vi "App - analyze RUS V6.vi"() -> ()   [LabVIEW 2018] (continued)
"file format"=enum."binary", "power(V)"=2.1, "Magn Field(T) "=0.0}, {"temperature"=20.054, "temperature str"="20.05400", "file path"=path "D:/Data/Ultrasound/LSCO/LSCO22__130814c/5_Cooling_2nd_try/September_2014/091714/20.05400K_500_2500_2.10000V_0.00000T_Sep17-2014__19-47-23_001_091714.bin", "last mod"=timestamp(3493842443 s since 1904-01-01), "file name str"="D:\\Data\\Ultrasound\\LSCO\\LSCO22__130814c\\5_Cooling_2nd_try\\September_2014\\091714\\20.05400K_500_2500_2.10000V_0.00000T_Sep17-2014__19-47-23_001_091714.bin", "mod time(min)"=58230707.38333333, "file format"=enum."binary", "power(V)"=2.1, "Magn Field(T) "=0.0}, {"temperature"=19.964, "temperature str"="19.96400", "file path"=path "D:/Data/Ultrasound/LSCO/LSCO22__130814c/5_Cooling_2nd_try/September_2014/091714/19.96400K_500_2500_2.10000V_0.00000T_Sep17-2014__19-48-42_001_091714.bin", "last mod"=timestamp(3493842522 s since 1904-01-01), "file name str"="D:\\Data\\Ultrasound\\LSCO\\LSCO22__130814c\\5_Cooling_2nd_try\\September_2014\\091714\\19.96400K_500_2500_2.10000V_0.00000T_Sep17-2014__19-48-42_001_091714.bin", "mod time(min)"=58230708.7, "file format"=enum."binary", "power(V)"=2.1, "Magn Field(T) "=0.0}, {"temperature"=19.857, "temperature str"="19.85700", "file path"=path "D:/Data/Ultrasound/LSCO/LSCO22__130814c/5_Cooling_2nd_try/September_2014/091714/19.85700K_500_2500_2.10000V_0.00000T_Sep17-2014__19-50-02_001_091714.bin", "last mod"=timestamp(3493842602 s since 1904-01-01), "file name str"="D:\\Data\\Ultrasound\\LSCO\\LSCO22__130814c\\5_Cooling_2nd_try\\September_2014\\091714\\19.85700K_500_2500_2.10000V_0.00000T_Sep17-2014__19-50-02_001_091714.bin", "mod time(min)"=58230710.03333333, "file format"=enum."binary", "power(V)"=2.1, "Magn Field(T) "=0.0}, {"temperature"=19.754, "temperature str"="19.75400", "file path"=path "D:/Data/Ultrasound/LSCO/LSCO22__130814c/5_Cooling_2nd_try/September_2014/091714/19.75400K_500_2500_2.10000V_0.00000T_Sep17-2014__19-51-21_001_091714.bin", "last mod"=timestamp(3493842681 s since 1904-01-01), "file name str"="D:\\Data\\Ultrasound\\LSCO\\LSCO22__130814c\\5_Cooling_2nd_try\\September_2014\\091714\\19.75400K_500_2500_2.10000V_0.00000T_Sep17-2014__19-51-21_001_091714.bin", "mod time(min)"=58230711.35, "file format"=enum."binary", "power(V)"=2.1, "Magn Field(T) "=0.0}, {"temperature"=19.658, "temperature str"="19.65800", "file path"=path "D:/Data/Ultrasound/LSCO/LSCO22__130814c/5_Cooling_2nd_try/September_2014/091714/19.65800K_500_2500_2.10000V_0.00000T_Sep17-2014__19-52-41_001_091714.bin", "last mod"=timestamp(3493842761 s since 1904-01-01), "file name str"="D:\\Data\\Ultrasound\\LSCO\\LSCO22__130814c\\5_Cooling_2nd_try\\September_2014\\091714\\19.65800K_500_2500_2.10000V_0.00000T_Sep17-2014__19-52-41_001_091714.bin", "mod time(min)"=58230712.68333333, "file format"=enum."binary", "power(V)"=2.1, "Magn Field(T) "=0.0}, {"temperature"=19.556, "temperature str"="19.55600", "file path"=path "D:/Data/Ultrasound/LSCO/LSCO22__130814c/5_Cooling_2nd_try/September_2014/091714/19.55600K_500_2500_2.10000V_0.00000T_Sep17-2014__19-54-00_001_091714.bin", "last mod"=timestamp(3493842840 s since 1904-01-01), "file name str"="D:\\Data\\Ultrasound\\LSCO\\LSCO22__130814c\\5_Cooling_2nd_try\\September_2014\\091714\\19.55600K_500_2500_2.10000V_0.00000T_Sep17-2014__19-54-00_001_091714.bin", "mod time(min)"=58230714.0, "file format"=enum."binary", "power(V)"=2.1, "Magn Field(T) "=0.0}, {"temperature"=19.452, "temperature str"="19.45200", "file path"=path "D:/Data/Ultrasound/LSCO/LSCO22__130814c/5_Cooling_2nd_try/September_2014/091714/19.45200K_500_2500_2.10000V_0.00000T_Sep17-2014__19-55-19_001_091714.bin", "last mod"=timestamp(3493842919 s since 1904-01-01), "file name str"="D:\\Data\\Ultrasound\\LSCO\\LSCO22__130814c\\5_Cooling_2nd_try\\September_2014\\091714\\19.45200K_500_2500_2.10000V_0.00000T_Sep17-2014__19-55-19_001_091714.bin", "mod time(min)"=58230715.31666667, "file format"=enum."binary", "power(V)"=2.1, "Magn Field(T) "=0.0}, {"temperature"=19.356, "temperature str"="19.35600", "file path"=path "D:/Data/Ultrasound/LSCO/LSCO22__130814c/5_Cooling_2nd_try/September_2014/091714/19.35600K_500_2500_2.10000V_0.00000T_Sep17-2014__19-56-39_001_091714.bin", "last mod"=timestamp(3493842999 s since 1904-01-01), "file name str"="D:\\Data\\Ultrasound\\LSCO\\LSCO22__130814c\\5_Cooling_2nd_try\\September_2014\\091714\\19.35600K_500_2500_2.10000V_0.00000T_Sep17-2014__19-56-39_001_091714.bin", "mod time(min)"=58230716.65, "file format"=enum."binary", "power(V)"=2.1, "Magn Field(T) "=0.0}, {"temperature"=19.258, "temperature str"="19.25800", "file path"=path "D:/Data/Ultrasound/LSCO/LSCO22__130814c/5_Cooling_2nd_try/September_2014/091714/19.25800K_500_2500_2.10000V_0.00000T_Sep17-2014__19-57-58_001_091714.bin", "last mod"=timestamp(3493843078 s since 1904-01-01), "file name str"="D:\\Data\\Ultrasound\\LSCO\\LSCO22__130814c\\5_Cooling_2nd_try\\September_2014\\091714\\19.25800K_500_2500_2.10000V_0.00000T_Sep17-2014__19-57-58_001_091714.bin", "mod time(min)"=58230717.96666667, "file format"=enum."binary", "power(V)"=2.1, "Magn Field(T) "=0.0}, {"temperature"=19.154, "temperature str"="19.15400", "file path"=path "D:/Data/Ultrasound/LSCO/LSCO22__130814c/5_Cooling_2nd_try/September_2014/091714/19.15400K_500_2500_2.10000V_0.00000T_Sep17-2014__19-59-17_001_091714.bin", "last mod"=timestamp(3493843157 s since 1904-01-01), "file name str"="D:\\Data\\Ultrasound\\LSCO\\LSCO22__130814c\\5_Cooling_2nd_try\\September_2014\\091714\\19.15400K_500_2500_2.10000V_0.00000T_Sep17-2014__19-59-17_001_091714.bin", "mod time(min)"=58230719.28333333, "file format"=enum."binary", "power(V)"=2.1, "Magn Field(T) "=0.0}, {"temperature"=19.054, "temperature str"="19.05400", "file path"=path "D:/Data/Ultrasound/LSCO/LSCO22__130814c/5_Cooling_2nd_try/September_2014/091714/19.05400K_500_2500_2.10000V_0.00000T_Sep17-2014__20-00-37_001_091714.bin", "last mod"=timestamp(3493843237 s since 1904-01-01), "file name str"="D:\\Data\\Ultrasound\\LSCO\\LSCO22__130814c\\5_Cooling_2nd_try\\September_2014\\091714\\19.05400K_500_2500_2.10000V_0.00000T_Sep17-2014__20-00-37_001_091714.bin", "mod time(min)"=58230720.61666667, "file format"=enum."binary", "power(V)"=2.1, "Magn Field(T) "=0.0}, {"temperature"=18.951, "temperature str"="18.95100", "file path"=path "D:/Data/Ultrasound/LSCO/LSCO22__130814c/5_Cooling_2nd_try/September_2014/091714/18.95100K_500_2500_2.10000V_0.00000T_Sep17-2014__20-01-56_001_091714.bin", "last mod"=timestamp(3493843316 s since 1904-01-01), "file name str"="D:\\Data\\Ultrasound\\LSCO\\LSCO22__130814c\\5_Cooling_2nd_try\\September_2014\\091714\\18.95100K_500_2500_2.10000V_0.00000T_Sep17-2014__20-01-56_001_091714.bin", "mod time(min)"=58230721.93333333, "file format"=enum."binary", "power(V)"=2.1, "Magn Field(T) "=0.0}, {"temperature"=18.852, "temperature str"="18.85200", "file path"=path "D:/Data/Ultrasound/LSCO/LSCO22__130814c/5_Cooling_2nd_try/September_2014/091714/18.85200K_500_2500_2.10000V_0.00000T_Sep17-2014__20-03-16_001_091714.bin", "last mod"=timestamp(3493843396 s since 1904-01-01), "file name str"="D:\\Data\\Ultrasound\\LSCO\\LSCO22__130814c\\5_Cooling_2nd_try\\September_2014\\091714\\18.85200K_500_2500_2.10000V_0.00000T_Sep17-2014__20-03-16_001_091714.bin", "mod time(min)"=58230723.266666666, "file format"=enum."binary", "power(V)"=2.1, "Magn Field(T) "=0.0}, {"temperature"=18.757, "temperature str"="18.75700", "file path"=path "D:/Data/Ultrasound/LSCO/LSCO22__130814c/5_Cooling_2nd_try/September_2014/091714/18.75700K_500_2500_2.10000V_0.00000T_Sep17-2014__20-04-35_001_091714.bin", "last mod"=timestamp(3493843475 s since 1904-01-01), "file name str"="D:\\Data\\Ultrasound\\LSCO\\LSCO22__130814c\\5_Cooling_2nd_try\\September_2014\\091714\\18.75700K_500_2500_2.10000V_0.00000T_Sep17-2014__20-04-35_001_091714.bin", "mod time(min)"=58230724.583333336, "file format"=enum."binary", "power(V)"=2.1, "Magn Field(T) "=0.0}, {"temperature"=18.649, "temperature str"="18.64900", "file path"=path "D:/Data/Ultrasound/LSCO/LSCO22__130814c/5_Cooling_2nd_try/September_2014/091714/18.64900K_500_2500_2.10000V_0.00000T_Sep17-2014__20-05-54_001_091714.bin", "last mod"=timestamp(3493843554 s since 1904-01-01), "file name str"="D:\\Data\\Ultrasound\\LSCO\\LSCO22__130814c\\5_Cooling_2nd_try\\September_2014\\091714\\18.64900K_500_2500_2.10000V_0.00000T_Sep17-2014__20-05-54_001_091714.bin", "mod time(min)"=58230725.9, "file format"=enum."binary", "power(V)"=2.1, "Magn Field(T) "=0.0}, {"temperature"=18.548, "temperature str"="18.54800", "file path"=path "D:/Data/Ultrasound/LSCO/LSCO22__130814c/5_Cooling_2nd_try/September_2014/091714/18.54800K_500_2500_2.10000V_0.00000T_Sep17-2014__20-07-14_001_091714.bin", "last mod"=timestamp(3493843634 s since 1904-01-01), "file name str"="D:\\Data\\Ultrasound\\LSCO\\LSCO22__130814c\\5_Cooling_2nd_try\\September_2014\\091714\\18.54800K_500_2500_2.10000V_0.00000T_Sep17-2014__20-07-14_001_091714.bin", "mod time(min)"=58230727.233333334, "file format"=enum."binary", "power(V)"=2.1, "Magn Field(T) "=0.0}, {"temperature"=18.451, "temperature str"="18.45100", "file path"=path "D:/Data/Ultrasound/LSCO/LSCO22__130814c/5_Cooling_2nd_try/September_2014/091714/18.45100K_500_2500_2.10000V_0.00000T_Sep17-2014__20-08-33_001_091714.bin", "last mod"=timestamp(3493843713 s since 1904-01-01), "file name str"="D:\\Data\\Ultrasound\\LSCO\\LSCO22__130814c\\5_Cooling_2nd_try\\September_2014\\091714\\18.45100K_500_2500_2.10000V_0.00000T_Sep17-2014__20-08-33_001_091714.bin", "mod time(min)"=58230728.55, "file format"=enum."binary", "power(V)"=2.1, "Magn Field(T) "=0.0}, {"temperature"=18.346, "temperature str"="18.34600", "file path"=path "D:/Data/Ultrasound/LSCO/LSCO22__130814c/5_Cooling_2nd_try/September_2014/091714/18.34600K_500_2500_2.10000V_0.00000T_Sep17-2014__20-09-53_001_091714.bin", "last mod"=timestamp(3493843793 s since 1904-01-01), "file name str"="D:\\Data\\Ultrasound\\LSCO\\LSCO22__130814c\\5_Cooling_2nd_try\\September_2014\\091714\\18.34600K_500_2500_2.10000V_0.00000T_Sep17-2014__20-09-53_001_091714.bin", "mod time(min)"=58230729.88333333, "file format"=enum."binary", "power(V)"=2.1, "Magn Field(T) "=0.0}, {"temperature"=18.245, "temperature str"="18.24500", "file path"=path "D:/Data/Ultrasound/LSCO/LSCO22__130814c/5_Cooling_2nd_try/September_2014/091714/18.24500K_500_2500_2.10000V_0.00000T_Sep17-2014__20-11-12_001_091714.bin", "last mod"=timestamp(3493843872 s since 1904-01-01), "file name str"="D:\\Data\\Ultrasound\\LSCO\\LSCO22__130814c\\5_Cooling_2nd_try\\September_2014\\091714\\18.24500K_500_2500_2.10000V_0.00000T_Sep17-2014__20-11-12_001_091714.bin", "mod time(min)"=58230731.2, "file format"=enum."binary", "power(V)"=2.1, "Magn Field(T) "=0.0}, {"temperature"=18.147, "temperature str"="18.14700", "file path"=path "D:/Data/Ultrasound/LSCO/LSCO22__130814c/5_Cooling_2nd_try/September_2014/091714/18.14700K_500_2500_2.10000V_0.00000T_Sep17-2014__20-12-31_001_091714.bin", "last mod"=timestamp(3493843951 s since 1904-01-01), "file name str"="D:\\Data\\Ultrasound\\LSCO\\LSCO22__130814c\\5_Cooling_2nd_try\\September_2014\\091714\\18.14700K_500_2500_2.10000V_0.00000T_Sep17-2014__20-12-31_001_091714.bin", "mod time(min)"=58230732.516666666, "file format"=enum."binary", "power(V)"=2.1, "Magn Field(T) "=0.0}, {"temperature"=18.042, "temperature str"="18.04200", "file path"=path "D:/Data/Ultrasound/LSCO/LSCO22__130814c/5_Cooling_2nd_try/September_2014/091714/18.04200K_500_2500_2.10000V_0.00000T_Sep17-2014__20-13-51_001_091714.bin", "last mod"=timestamp(3493844031 s since 1904-01-01), "file name str"="D:\\Data\\Ultrasound\\LSCO\\LSCO22__130814c\\5_Cooling_2nd_try\\September_2014\\091714\\18.04200K_500_2500_2.10000V_0.00000T_Sep17-2014__20-13-51_001_091714.bin", "mod time(min)"=58230733.85, "file format"=enum."binary", "power(V)"=2.1, "Magn Field(T) "=0.0}, {"temperature"=17.951, "temperature str"="17.95100", "file path"=path "D:/Data/Ultrasound/LSCO/LSCO22__130814c/5_Cooling_2nd_try/September_2014/091714/17.95100K_500_2500_2.10000V_0.00000T_Sep17-2014__20-15-10_001_091714.bin", "last mod"=timestamp(3493844110 s since 1904-01-01), "file name str"="D:\\Data\\Ultrasound\\LSCO\\LSCO22__130814c\\5_Cooling_2nd_try\\September_2014\\091714\\17.95100K_500_2500_2.10000V_0.00000T_Sep17-2014__20-15-10_001_091714.bin", "mod time(min)"=58230735.166666664, "file format"=enum."binary", "power(V)"=2.1, "Magn Field(T) "=0.0}, {"temperature"=17.844, "temperature str"="17.84400", "file path"=path "D:/Data/Ultrasound/LSCO/LSCO22__130814c/5_Cooling_2nd_try/September_2014/091714/17.84400K_500_2500_2.10000V_0.00000T_Sep17-2014__20-16-29_001_091714.bin", "last mod"=timestamp(3493844189 s since 1904-01-01), "file name str"="D:\\Data\\Ultrasound\\LSCO\\LSCO22__130814c\\5_Cooling_2nd_try\\September_2014\\091714\\17.84400K_500_2500_2.10000V_0.00000T_Sep17-2014__20-16-29_001_091714.bin", "mod time(min)"=58230736.483333334, "file format"=enum."binary", "power(V)"=2.1, "Magn Field(T) "=0.0}, {"temperature"=17.735, "temperature str"="17.73500", "file path"=path "D:/Data/Ultrasound/LSCO/LSCO22__130814c/5_Cooling_2nd_try/September_2014/091714/17.73500K_500_2500_2.10000V_0.00000T_Sep17-2014__20-17-49_001_091714.bin", "last mod"=timestamp(3493844269 s since 1904-01-01), "file name str"="D:\\Data\\Ultrasound\\LSCO\\LSCO22__130814c\\5_Cooling_2nd_try\\September_2014\\091714\\17.73500K_500_2500_2.10000V_0.00000T_Sep17-2014__20-17-49_001_091714.bin", "mod time(min)"=58230737.81666667, "file format"=enum."binary", "power(V)"=2.1, "Magn Field(T) "=0.0}, {"temperature"=17.643, "temperature str"="17.64300", "file path"=path "D:/Data/Ultrasound/LSCO/LSCO22__130814c/5_Cooling_2nd_try/September_2014/091714/17.64300K_500_2500_2.10000V_0.00000T_Sep17-2014__20-19-08_001_091714.bin", "last mod"=timestamp(3493844348 s since 1904-01-01), "file name str"="D:\\Data\\Ultrasound\\LSCO\\LSCO22__130814c\\5_Cooling_2nd_try\\September_2014\\091714\\17.64300K_500_2500_2.10000V_0.00000T_Sep17-2014__20-19-08_001_091714.bin", "mod time(min)"=58230739.13333333, "file format"=enum."binary", "power(V)"=2.1, "Magn Field(T) "=0.0}, {"temperature"=17.54, "temperature str"="17.54000", "file path"=path "D:/Data/Ultrasound/LSCO/LSCO22__130814c/5_Cooling_2nd_try/September_2014/091714/17.54000K_500_2500_2.10000V_0.00000T_Sep17-2014__20-20-28_001_091714.bin", "last mod"=timestamp(3493844428 s since 1904-01-01), "file name str"="D:\\Data\\Ultrasound\\LSCO\\LSCO22__130814c\\5_Cooling_2nd_try\\September_2014\\091714\\17.54000K_500_2500_2.10000V_0.00000T_Sep17-2014__20-20-28_001_091714.bin", "mod time(min)"=58230740.46666667, "file format"=enum."binary", "power(V)"=2.1, "Magn Field(T) "=0.0}, {"temperature"=17.438, "temperature str"="17.43800", "file path"=path "D:/Data/Ultrasound/LSCO/LSCO22__130814c/5_Cooling_2nd_try/September_2014/091714/17.43800K_500_2500_2.10000V_0.00000T_Sep17-2014__20-21-47_001_091714.bin", "last mod"=timestamp(3493844507 s since 1904-01-01), "file name str"="D:\\Data\\Ultrasound\\LSCO\\LSCO22__130814c\\5_Cooling_2nd_try\\September_2014\\091714\\17.43800K_500_2500_2.10000V_0.00000T_Sep17-2014__20-21-47_001_091714.bin", "mod time(min)"=58230741.78333333, "file format"=enum."binary", "power(V)"=2.1, "Magn Field(T) "=0.0}, {"temperature"=17.338, "temperature str"="17.33800", "file path"=path "D:/Data/Ultrasound/LSCO/LSCO22__130814c/5_Cooling_2nd_try/September_2014/091714/17.33800K_500_2500_2.10000V_0.00000T_Sep17-2014__20-23-06_001_091714.bin", "last mod"=timestamp(3493844586 s since 1904-01-01), "file name str"="D:\\Data\\Ultrasound\\LSCO\\LSCO22__130814c\\5_Cooling_2nd_try\\September_2014\\091714\\17.33800K_500_2500_2.10000V_0.00000T_Sep17-2014__20-23-06_001_091714.bin", "mod time(min)"=58230743.1, "file format"=enum."binary", "power(V)"=2.1, "Magn Field(T) "=0.0}, {"temperature"=17.235, "temperature str"="17.23500", "file path"=path "D:/Data/Ultrasound/LSCO/LSCO22__130814c/5_Cooling_2nd_try/September_2014/091714/17.23500K_500_2500_2.10000V_0.00000T_Sep17-2014__20-24-26_001_091714.bin", "last mod"=timestamp(3493844666 s since 1904-01-01), "file name str"="D:\\Data\\Ultrasound\\LSCO\\LSCO22__130814c\\5_Cooling_2nd_try\\September_2014\\091714\\17.23500K_500_2500_2.10000V_0.00000T_Sep17-2014__20-24-26_001_091714.bin", "mod time(min)"=58230744.43333333, "file format"=enum."binary", "power(V)"=2.1, "Magn Field(T) "=0.0}, {"temperature"=17.133, "temperature str"="17.13300", "file path"=path "D:/Data/Ultrasound/LSCO/LSCO22__130814c/5_Cooling_2nd_try/September_2014/091714/17.13300K_500_2500_2.10000V_0.00000T_Sep17-2014__20-25-45_001_091714.bin", "last mod"=timestamp(3493844745 s since 1904-01-01), "file name str"="D:\\Data\\Ultrasound\\LSCO\\LSCO22__130814c\\5_Cooling_2nd_try\\September_2014\\091714\\17.13300K_500_2500_2.10000V_0.00000T_Sep17-2014__20-25-45_001_091714.bin", "mod time(min)"=58230745.75, "file format"=enum."binary", "power(V)"=2.1, "Magn Field(T) "=0.0}, {"temperature"=17.034, "temperature str"="17.03400", "file path"=path "D:/Data/Ultrasound/LSCO/LSCO22__130814c/5_Cooling_2nd_try/September_2014/091714/17.03400K_500_2500_2.10000V_0.00000T_Sep17-2014__20-27-04_001_091714.bin", "last mod"=timestamp(3493844824 s since 1904-01-01), "file name str"="D:\\Data\\Ultrasound\\LSCO\\LSCO22__130814c\\5_Cooling_2nd_try\\September_2014\\091714\\17.03400K_500_2500_2.10000V_0.00000T_Sep17-2014__20-27-04_001_091714.bin", "mod time(min)"=58230747.06666667, "file format"=enum."binary", "power(V)"=2.1, "Magn Field(T) "=0.0}, {"temperature"=16.936, "temperature str"="16.93600", "file path"=path "D:/Data/Ultrasound/LSCO/LSCO22__130814c/5_Cooling_2nd_try/September_2014/091714/16.93600K_500_2500_2.10000V_0.00000T_Sep17-2014__20-28-24_001_091714.bin", "last mod"=timestamp(3493844904 s since 1904-01-01), "file name str"="D:\\Data\\Ultrasound\\LSCO\\LSCO22__130814c\\5_Cooling_2nd_try\\September_2014\\091714\\16.93600K_500_2500_2.10000V_0.00000T_Sep17-2014__20-28-24_001_091714.bin", "mod time(min)"=58230748.4, "file format"=enum."binary", "power(V)"=2.1, "Magn Field(T) "=0.0}, {"temperature"=16.831, "temperature str"="16.83100", "file path"=path "D:/Data/Ultrasound/LSCO/LSCO22__130814c/5_Cooling_2nd_try/September_2014/091714/16.83100K_500_2500_2.10000V_0.00000T_Sep17-2014__20-29-43_001_091714.bin", "last mod"=timestamp(3493844983 s since 1904-01-01), "file name str"="D:\\Data\\Ultrasound\\LSCO\\LSCO22__130814c\\5_Cooling_2nd_try\\September_2014\\091714\\16.83100K_500_2500_2.10000V_0.00000T_Sep17-2014__20-29-43_001_091714.bin", "mod time(min)"=58230749.71666667, "file format"=enum."binary", "power(V)"=2.1, "Magn Field(T) "=0.0}, {"temperature"=16.732, "temperature str"="16.73200", "file path"=path "D:/Data/Ultrasound/LSCO/LSCO22__130814c/5_Cooling_2nd_try/September_2014/091714/16.73200K_500_2500_2.10000V_0.00000T_Sep17-2014__20-31-03_001_091714.bin", "last mod"=timestamp(3493845063 s since 1904-01-01), "file name str"="D:\\Data\\Ultrasound\\LSCO\\LSCO22__130814c\\5_Cooling_2nd_try\\September_2014\\091714\\16.73200K_500_2500_2.10000V_0.00000T_Sep17-2014__20-31-03_001_091714.bin", "mod time(min)"=58230751.05, "file format"=enum."binary", "power(V)"=2.1, "Magn Field(T) "=0.0}, {"temperature"=16.631, "temperature str"="16.63100", "file path"=path "D:/Data/Ultrasound/LSCO/LSCO22__130814c/5_Cooling_2nd_try/September_2014/091714/16.63100K_500_2500_2.10000V_0.00000T_Sep17-2014__20-32-22_001_091714.bin", "last mod"=timestamp(3493845142 s since 1904-01-01), "file name str"="D:\\Data\\Ultrasound\\LSCO\\LSCO22__130814c\\5_Cooling_2nd_try\\September_2014\\091714\\16.63100K_500_2500_2.10000V_0.00000T_Sep17-2014__20-32-22_001_091714.bin", "mod time(min)"=58230752.36666667, "file format"=enum."binary", "power(V)"=2.1, "Magn Field(T) "=0.0}, {"temperature"=16.524, "temperature str"="16.52400", "file path"=path "D:/Data/Ultrasound/LSCO/LSCO22__130814c/5_Cooling_2nd_try/September_2014/091714/16.52400K_500_2500_2.10000V_0.00000T_Sep17-2014__20-33-41_001_091714.bin", "last mod"=timestamp(3493845221 s since 1904-01-01), "file name str"="D:\\Data\\Ultrasound\\LSCO\\LSCO22__130814c\\5_Cooling_2nd_try\\September_2014\\091714\\16.52400K_500_2500_2.10000V_0.00000T_Sep17-2014__20-33-41_001_091714.bin", "mod time(min)"=58230753.68333333, "file format"=enum."binary", "power(V)"=2.1, "Magn Field(T) "=0.0}, {"temperature"=16.433, "temperature str"="16.43300", "file path"=path "D:/Data/Ultrasound/LSCO/LSCO22__130814c/5_Cooling_2nd_try/September_2014/091714/16.43300K_500_2500_2.10000V_0.00000T_Sep17-2014__20-35-01_001_091714.bin", "last mod"=timestamp(3493845301 s since 1904-01-01), "file name str"="D:\\Data\\Ultrasound\\LSCO\\LSCO22__130814c\\5_Cooling_2nd_try\\September_2014\\091714\\16.43300K_500_2500_2.10000V_0.00000T_Sep17-2014__20-35-01_001_091714.bin", "mod time(min)"=58230755.016666666, "file format"=enum."binary", "power(V)"=2.1, "Magn Field(T) "=0.0}, {"temperature"=16.322, "temperature str"="16.32200", "file path"=path "D:/Data/Ultrasound/LSCO/LSCO22__130814c/5_Cooling_2nd_try/September_2014/091714/16.32200K_500_2500_2.10000V_0.00000T_Sep17-2014__20-36-20_001_091714.bin", "last mod"=timestamp(3493845380 s since 1904-01-01), "file name str"="D:\\Data\\Ultrasound\\LSCO\\LSCO22__130814c\\5_Cooling_2nd_try\\September_2014\\091714\\16.32200K_500_2500_2.10000V_0.00000T_Sep17-2014__20-36-20_001_091714.bin", "mod time(min)"=58230756.333333336, "file format"=enum."binary", "power(V)"=2.1, "Magn Field(T) "=0.0}, {"temperature"=16.223, "temperature str"="16.22300", "file path"=path "D:/Data/Ultrasound/LSCO/LSCO22__130814c/5_Cooling_2nd_try/September_2014/091714/16.22300K_500_2500_2.10000V_0.00000T_Sep17-2014__20-37-40_001_091714.bin", "last mod"=timestamp(3493845460 s since 1904-01-01), "file name str"="D:\\Data\\Ultrasound\\LSCO\\LSCO22__130814c\\5_Cooling_2nd_try\\September_2014\\091714\\16.22300K_500_2500_2.10000V_0.00000T_Sep17-2014__20-37-40_001_091714.bin", "mod time(min)"=58230757.666666664, "file format"=enum."binary", "power(V)"=2.1, "Magn Field(T) "=0.0}, {"temperature"=16.128, "temperature str"="16.12800", "file path"=path "D:/Data/Ultrasound/LSCO/LSCO22__130814c/5_Cooling_2nd_try/September_2014/091714/16.12800K_500_2500_2.10000V_0.00000T_Sep17-2014__20-38-59_001_091714.bin", "last mod"=timestamp(3493845539 s since 1904-01-01), "file name str"="D:\\Data\\Ultrasound\\LSCO\\LSCO22__130814c\\5_Cooling_2nd_try\\September_2014\\091714\\16.12800K_500_2500_2.10000V_0.00000T_Sep17-2014__20-38-59_001_091714.bin", "mod time(min)"=58230758.983333334, "file format"=enum."binary", "power(V)"=2.1, "Magn Field(T) "=0.0}, {"temperature"=16.024, "temperature str"="16.02400", "file path"=path "D:/Data/Ultrasound/LSCO/LSCO22__130814c/5_Cooling_2nd_try/September_2014/091714/16.02400K_500_2500_2.10000V_0.00000T_Sep17-2014__20-40-18_001_091714.bin", "last mod"=timestamp(3493845618 s since 1904-01-01), "file name str"="D:\\Data\\Ultrasound\\LSCO\\LSCO22__130814c\\5_Cooling_2nd_try\\September_2014\\091714\\16.02400K_500_2500_2.10000V_0.00000T_Sep17-2014__20-40-18_001_091714.bin", "mod time(min)"=58230760.3, "file format"=enum."binary", "power(V)"=2.1, "Magn Field(T) "=0.0}, {"temperature"=15.924, "temperature str"="15.92400", "file path"=path "D:/Data/Ultrasound/LSCO/LSCO22__130814c/5_Cooling_2nd_try/September_2014/091714/15.92400K_500_2500_2.10000V_0.00000T_Sep17-2014__20-41-38_001_091714.bin", "last mod"=timestamp(3493845698 s since 1904-01-01), "file name str"="D:\\Data\\Ultrasound\\LSCO\\LSCO22__130814c\\5_Cooling_2nd_try\\September_2014\\091714\\15.92400K_500_2500_2.10000V_0.00000T_Sep17-2014__20-41-38_001_091714.bin", "mod time(min)"=58230761.63333333, "file format"=enum."binary", "power(V)"=2.1, "Magn Field(T) "=0.0}, {"temperature"=15.82, "temperature str"="15.82000", "file path"=path "D:/Data/Ultrasound/LSCO/LSCO22__130814c/5_Cooling_2nd_try/September_2014/091714/15.82000K_500_2500_2.10000V_0.00000T_Sep17-2014__20-42-57_001_091714.bin", "last mod"=timestamp(3493845777 s since 1904-01-01), "file name str"="D:\\Data\\Ultrasound\\LSCO\\LSCO22__130814c\\5_Cooling_2nd_try\\September_2014\\091714\\15.82000K_500_2500_2.10000V_0.00000T_Sep17-2014__20-42-57_001_091714.bin", "mod time(min)"=58230762.95, "file format"=enum."binary", "power(V)"=2.1, "Magn Field(T) "=0.0}, {"temperature"=15.723, "temperature str"="15.72300", "file path"=path "D:/Data/Ultrasound/LSCO/LSCO22__130814c/5_Cooling_2nd_try/September_2014/091714/15.72300K_500_2500_2.10000V_0.00000T_Sep17-2014__20-44-16_001_091714.bin", "last mod"=timestamp(3493845856 s since 1904-01-01), "file name str"="D:\\Data\\Ultrasound\\LSCO\\LSCO22__130814c\\5_Cooling_2nd_try\\September_2014\\091714\\15.72300K_500_2500_2.10000V_0.00000T_Sep17-2014__20-44-16_001_091714.bin", "mod time(min)"=58230764.266666666, "file format"=enum."binary", "power(V)"=2.1, "Magn Field(T) "=0.0}, {"temperature"=15.622, "temperature str"="15.62200", "file path"=path "D:/Data/Ultrasound/LSCO/LSCO22__130814c/5_Cooling_2nd_try/September_2014/091714/15.62200K_500_2500_2.10000V_0.00000T_Sep17-2014__20-45-36_001_091714.bin", "last mod"=timestamp(3493845936 s since 1904-01-01), "file name str"="D:\\Data\\Ultrasound\\LSCO\\LSCO22__130814c\\5_Cooling_2nd_try\\September_2014\\091714\\15.62200K_500_2500_2.10000V_0.00000T_Sep17-2014__20-45-36_001_091714.bin", "mod time(min)"=58230765.6, "file format"=enum."binary", "power(V)"=2.1, "Magn Field(T) "=0.0}, {"temperature"=15.52, "temperature str"="15.52000", "file path"=path "D:/Data/Ultrasound/LSCO/LSCO22__130814c/5_Cooling_2nd_try/September_2014/091714/15.52000K_500_2500_2.10000V_0.00000T_Sep17-2014__20-46-55_001_091714.bin", "last mod"=timestamp(3493846015 s since 1904-01-01), "file name str"="D:\\Data\\Ultrasound\\LSCO\\LSCO22__130814c\\5_Cooling_2nd_try\\September_2014\\091714\\15.52000K_500_2500_2.10000V_0.00000T_Sep17-2014__20-46-55_001_091714.bin", "mod time(min)"=58230766.916666664, "file format"=enum."binary", "power(V)"=2.1, "Magn Field(T) "=0.0}, {"temperature"=15.419, "temperature str"="15.41900", "file path"=path "D:/Data/Ultrasound/LSCO/LSCO22__130814c/5_Cooling_2nd_try/September_2014/091714/15.41900K_500_2500_2.10000V_0.00000T_Sep17-2014__20-48-15_001_091714.bin", "last mod"=timestamp(3493846095 s since 1904-01-01), "file name str"="D:\\Data\\Ultrasound\\LSCO\\LSCO22__130814c\\5_Cooling_2nd_try\\September_2014\\091714\\15.41900K_500_2500_2.10000V_0.00000T_Sep17-2014__20-48-15_001_091714.bin", "mod time(min)"=58230768.25, "file format"=enum."binary", "power(V)"=2.1, "Magn Field(T) "=0.0}, {"temperature"=15.33, "temperature str"="15.33000", "file path"=path "D:/Data/Ultrasound/LSCO/LSCO22__130814c/5_Cooling_2nd_try/September_2014/091714/15.33000K_500_2500_2.10000V_0.00000T_Sep17-2014__20-49-34_001_091714.bin", "last mod"=timestamp(3493846174 s since 1904-01-01), "file name str"="D:\\Data\\Ultrasound\\LSCO\\LSCO22__130814c\\5_Cooling_2nd_try\\September_2014\\091714\\15.33000K_500_2500_2.10000V_0.00000T_Sep17-2014__20-49-34_001_091714.bin", "mod time(min)"=58230769.56666667, "file format"=enum."binary", "power(V)"=2.1, "Magn Field(T) "=0.0}, {"temperature"=15.223, "temperature str"="15.22300", "file path"=path "D:/Data/Ultrasound/LSCO/LSCO22__130814c/5_Cooling_2nd_try/September_2014/091714/15.22300K_500_2500_2.10000V_0.00000T_Sep17-2014__20-50-53_001_091714.bin", "last mod"=timestamp(3493846253 s since 1904-01-01), "file name str"="D:\\Data\\Ultrasound\\LSCO\\LSCO22__130814c\\5_Cooling_2nd_try\\September_2014\\091714\\15.22300K_500_2500_2.10000V_0.00000T_Sep17-2014__20-50-53_001_091714.bin", "mod time(min)"=58230770.88333333, "file format"=enum."binary", "power(V)"=2.1, "Magn Field(T) "=0.0}, {"temperature"=15.166, "temperature str"="15.16600", "file path"=path "D:/Data/Ultrasound/LSCO/LSCO22__130814c/5_Cooling_2nd_try/September_2014/091714/15.16600K_500_2500_2.10000V_0.00000T_Sep17-2014__20-52-13_001_091714.bin", "last mod"=timestamp(3493846333 s since 1904-01-01), "file name str"="D:\\Data\\Ultrasound\\LSCO\\LSCO22__130814c\\5_Cooling_2nd_try\\September_2014\\091714\\15.16600K_500_2500_2.10000V_0.00000T_Sep17-2014__20-52-13_001_091714.bin", "mod time(min)"=58230772.21666667, "file format"=enum."binary", "power(V)"=2.1, "Magn Field(T) "=0.0}, {"temperature"=15.139, "temperature str"="15.13900", "file path"=path "D:/Data/Ultrasound/LSCO/LSCO22__130814c/5_Cooling_2nd_try/September_2014/091714/15.13900K_500_2500_2.10000V_0.00000T_Sep17-2014__20-53-32_001_091714.bin", "last mod"=timestamp(3493846412 s since 1904-01-01), "file name str"="D:\\Data\\Ultrasound\\LSCO\\LSCO22__130814c\\5_Cooling_2nd_try\\September_2014\\091714\\15.13900K_500_2500_2.10000V_0.00000T_Sep17-2014__20-53-32_001_091714.bin", "mod time(min)"=58230773.53333333, "file format"=enum."binary", "power(V)"=2.1, "Magn Field(T) "=0.0}, {"temperature"=15.12, "temperature str"="15.12000", "file path"=path "D:/Data/Ultrasound/LSCO/LSCO22__130814c/5_Cooling_2nd_try/September_2014/091714/15.12000K_500_2500_2.10000V_0.00000T_Sep17-2014__20-54-52_001_091714.bin", "last mod"=timestamp(3493846492 s since 1904-01-01), "file name str"="D:\\Data\\Ultrasound\\LSCO\\LSCO22__130814c\\5_Cooling_2nd_try\\September_2014\\091714\\15.12000K_500_2500_2.10000V_0.00000T_Sep17-2014__20-54-52_001_091714.bin", "mod time(min)"=58230774.86666667, "file format"=enum."binary", "power(V)"=2.1, "Magn Field(T) "=0.0}, {"temperature"=15.102, "temperature str"="15.10200", "file path"=path "D:/Data/Ultrasound/LSCO/LSCO22__130814c/5_Cooling_2nd_try/September_2014/091714/15.10200K_500_2500_2.10000V_0.00000T_Sep17-2014__20-56-11_001_091714.bin", "last mod"=timestamp(3493846571 s since 1904-01-01), "file name str"="D:\\Data\\Ultrasound\\LSCO\\LSCO22__130814c\\5_Cooling_2nd_try\\September_2014\\091714\\15.10200K_500_2500_2.10000V_0.00000T_Sep17-2014__20-56-11_001_091714.bin", "mod time(min)"=58230776.18333333, "file format"=enum."binary", "power(V)"=2.1, "Magn Field(T) "=0.0}, {"temperature"=15.094, "temperature str"="15.09400", "file path"=path "D:/Data/Ultrasound/LSCO/LSCO22__130814c/5_Cooling_2nd_try/September_2014/091714/15.09400K_500_2500_2.10000V_0.00000T_Sep17-2014__20-57-30_001_091714.bin", "last mod"=timestamp(3493846650 s since 1904-01-01), "file name str"="D:\\Data\\Ultrasound\\LSCO\\LSCO22__130814c\\5_Cooling_2nd_try\\September_2014\\091714\\15.09400K_500_2500_2.10000V_0.00000T_Sep17-2014__20-57-30_001_091714.bin", "mod time(min)"=58230777.5, "file format"=enum."binary", "power(V)"=2.1, "Magn Field(T) "=0.0}, {"temperature"=15.075, "temperature str"="15.07500", "file path"=path "D:/Data/Ultrasound/LSCO/LSCO22__130814c/5_Cooling_2nd_try/September_2014/091714/15.07500K_500_2500_2.10000V_0.00000T_Sep17-2014__20-58-50_001_091714.bin", "last mod"=timestamp(3493846730 s since 1904-01-01), "file name str"="D:\\Data\\Ultrasound\\LSCO\\LSCO22__130814c\\5_Cooling_2nd_try\\September_2014\\091714\\15.07500K_500_2500_2.10000V_0.00000T_Sep17-2014__20-58-50_001_091714.bin", "mod time(min)"=58230778.833333336, "file format"=enum."binary", "power(V)"=2.1, "Magn Field(T) "=0.0}, {"temperature"=15.065, "temperature str"="15.06500", "file path"=path "D:/Data/Ultrasound/LSCO/LSCO22__130814c/5_Cooling_2nd_try/September_2014/091714/15.06500K_500_2500_2.10000V_0.00000T_Sep17-2014__21-00-09_001_091714.bin", "last mod"=timestamp(3493846809 s since 1904-01-01), "file name str"="D:\\Data\\Ultrasound\\LSCO\\LSCO22__130814c\\5_Cooling_2nd_try\\September_2014\\091714\\15.06500K_500_2500_2.10000V_0.00000T_Sep17-2014__21-00-09_001_091714.bin", "mod time(min)"=58230780.15, "file format"=enum."binary", "power(V)"=2.1, "Magn Field(T) "=0.0}, {"temperature"=15.054, "temperature str"="15.05400", "file path"=path "D:/Data/Ultrasound/LSCO/LSCO22__130814c/5_Cooling_2nd_try/September_2014/091714/15.05400K_500_2500_2.10000V_0.00000T_Sep17-2014__21-01-28_001_091714.bin", "last mod"=timestamp(3493846888 s since 1904-01-01), "file name str"="D:\\Data\\Ultrasound\\LSCO\\LSCO22__130814c\\5_Cooling_2nd_try\\September_2014\\091714\\15.05400K_500_2500_2.10000V_0.00000T_Sep17-2014__21-01-28_001_091714.bin", "mod time(min)"=58230781.46666667, "file format"=enum."binary", "power(V)"=2.1, "Magn Field(T) "=0.0}, {"temperature"=15.042, "temperature str"="15.04200", "file path"=path "D:/Data/Ultrasound/LSCO/LSCO22__130814c/5_Cooling_2nd_try/September_2014/091714/15.04200K_500_2500_2.10000V_0.00000T_Sep17-2014__21-02-48_001_091714.bin", "last mod"=timestamp(3493846968 s since 1904-01-01), "file name str"="D:\\Data\\Ultrasound\\LSCO\\LSCO22__130814c\\5_Cooling_2nd_try\\September_2014\\091714\\15.04200K_500_2500_2.10000V_0.00000T_Sep17-2014__21-02-48_001_091714.bin", "mod time(min)"=58230782.8, "file format"=enum."binary", "power(V)"=2.1, "Magn Field(T) "=0.0}, {"temperature"=15.031, "temperature str"="15.03100", "file path"=path "D:/Data/Ultrasound/LSCO/LSCO22__130814c/5_Cooling_2nd_try/September_2014/091714/15.03100K_500_2500_2.10000V_0.00000T_Sep17-2014__21-04-07_001_091714.bin", "last mod"=timestamp(3493847047 s since 1904-01-01), "file name str"="D:\\Data\\Ultrasound\\LSCO\\LSCO22__130814c\\5_Cooling_2nd_try\\September_2014\\091714\\15.03100K_500_2500_2.10000V_0.00000T_Sep17-2014__21-04-07_001_091714.bin", "mod time(min)"=58230784.11666667, "file format"=enum."binary", "power(V)"=2.1, "Magn Field(T) "=0.0}, {"temperature"=15.023, "temperature str"="15.02300", "file path"=path "D:/Data/Ultrasound/LSCO/LSCO22__130814c/5_Cooling_2nd_try/September_2014/091714/15.02300K_500_2500_2.10000V_0.00000T_Sep17-2014__21-05-27_001_091714.bin", "last mod"=timestamp(3493847127 s since 1904-01-01), "file name str"="D:\\Data\\Ultrasound\\LSCO\\LSCO22__130814c\\5_Cooling_2nd_try\\September_2014\\091714\\15.02300K_500_2500_2.10000V_0.00000T_Sep17-2014__21-05-27_001_091714.bin", "mod time(min)"=58230785.45, "file format"=enum."binary", "power(V)"=2.1, "Magn Field(T) "=0.0}, {"temperature"=15.011, "temperature str"="15.01100", "file path"=path "D:/Data/Ultrasound/LSCO/LSCO22__130814c/5_Cooling_2nd_try/September_2014/091714/15.01100K_500_2500_2.10000V_0.00000T_Sep17-2014__21-06-46_001_091714.bin", "last mod"=timestamp(3493847206 s since 1904-01-01), "file name str"="D:\\Data\\Ultrasound\\LSCO\\LSCO22__130814c\\5_Cooling_2nd_try\\September_2014\\091714\\15.01100K_500_2500_2.10000V_0.00000T_Sep17-2014__21-06-46_001_091714.bin", "mod time(min)"=58230786.766666666, "file format"=enum."binary", "power(V)"=2.1, "Magn Field(T) "=0.0}, {"temperature"=15.012, "temperature str"="15.01200", "file path"=path "D:/Data/Ultrasound/LSCO/LSCO22__130814c/5_Cooling_2nd_try/September_2014/091714/15.01200K_500_2500_2.10000V_0.00000T_Sep17-2014__21-08-05_001_091714.bin", "last mod"=timestamp(3493847285 s since 1904-01-01), "file name str"="D:\\Data\\Ultrasound\\LSCO\\LSCO22__130814c\\5_Cooling_2nd_try\\September_2014\\091714\\15.01200K_500_2500_2.10000V_0.00000T_Sep17-2014__21-08-05_001_091714.bin", "mod time(min)"=58230788.083333336, "file format"=enum."binary", "power(V)"=2.1, "Magn Field(T) "=0.0}, {"temperature"=15.016, "temperature str"="15.01600", "file path"=path "D:/Data/Ultrasound/LSCO/LSCO22__130814c/5_Cooling_2nd_try/September_2014/091714/15.01600K_500_2500_2.10000V_0.00000T_Sep17-2014__21-09-25_001_091714.bin", "last mod"=timestamp(3493847365 s since 1904-01-01), "file name str"="D:\\Data\\Ultrasound\\LSCO\\LSCO22__130814c\\5_Cooling_2nd_try\\September_2014\\091714\\15.01600K_500_2500_2.10000V_0.00000T_Sep17-2014__21-09-25_001_091714.bin", "mod time(min)"=58230789.416666664, "file format"=enum."binary", "power(V)"=2.1, "Magn Field(T) "=0.0}, {"temperature"=15.007, "temperature str"="15.00700", "file path"=path "D:/Data/Ultrasound/LSCO/LSCO22__130814c/5_Cooling_2nd_try/September_2014/091714/15.00700K_500_2500_2.10000V_0.00000T_Sep17-2014__21-10-44_001_091714.bin", "last mod"=timestamp(3493847444 s since 1904-01-01), "file name str"="D:\\Data\\Ultrasound\\LSCO\\LSCO22__130814c\\5_Cooling_2nd_try\\September_2014\\091714\\15.00700K_500_2500_2.10000V_0.00000T_Sep17-2014__21-10-44_001_091714.bin", "mod time(min)"=58230790.733333334, "file format"=enum."binary", "power(V)"=2.1, "Magn Field(T) "=0.0}, {"temperature"=15.003, "temperature str"="15.00300", "file path"=path "D:/Data/Ultrasound/LSCO/LSCO22__130814c/5_Cooling_2nd_try/September_2014/091714/15.00300K_500_2500_2.10000V_0.00000T_Sep17-2014__21-12-03_001_091714.bin", "last mod"=timestamp(3493847523 s since 1904-01-01), "file name str"="D:\\Data\\Ultrasound\\LSCO\\LSCO22__130814c\\5_Cooling_2nd_try\\September_2014\\091714\\15.00300K_500_2500_2.10000V_0.00000T_Sep17-2014__21-12-03_001_091714.bin", "mod time(min)"=58230792.05, "file format"=enum."binary", "power(V)"=2.1, "Magn Field(T) "=0.0}, {"temperature"=14.997, "temperature str"="14.99700", "file path"=path "D:/Data/Ultrasound/LSCO/LSCO22__130814c/5_Cooling_2nd_try/September_2014/091714/14.99700K_500_2500_2.10000V_0.00000T_Sep17-2014__21-13-23_001_091714.bin", "last mod"=timestamp(3493847603 s since 1904-01-01), "file name str"="D:\\Data\\Ultrasound\\LSCO\\LSCO22__130814c\\5_Cooling_2nd_try\\September_2014\\091714\\14.99700K_500_2500_2.10000V_0.00000T_Sep17-2014__21-13-23_001_091714.bin", "mod time(min)"=58230793.38333333, "file format"=enum."binary", "power(V)"=2.1, "Magn Field(T) "=0.0}, {"temperature"=14.985, "temperature str"="14.98500", "file path"=path "D:/Data/Ultrasound/LSCO/LSCO22__130814c/5_Cooling_2nd_try/September_2014/091714/14.98500K_500_2500_2.10000V_0.00000T_Sep17-2014__21-14-42_001_091714.bin", "last mod"=timestamp(3493847682 s since 1904-01-01), "file name str"="D:\\Data\\Ultrasound\\LSCO\\LSCO22__130814c\\5_Cooling_2nd_try\\September_2014\\091714\\14.98500K_500_2500_2.10000V_0.00000T_Sep17-2014__21-14-42_001_091714.bin", "mod time(min)"=58230794.7, "file format"=enum."binary", "power(V)"=2.1, "Magn Field(T) "=0.0}, {"temperature"=14.981, "temperature str"="14.98100", "file path"=path "D:/Data/Ultrasound/LSCO/LSCO22__130814c/5_Cooling_2nd_try/September_2014/091714/14.98100K_500_2500_2.10000V_0.00000T_Sep17-2014__21-16-02_001_091714.bin", "last mod"=timestamp(3493847762 s since 1904-01-01), "file name str"="D:\\Data\\Ultrasound\\LSCO\\LSCO22__130814c\\5_Cooling_2nd_try\\September_2014\\091714\\14.98100K_500_2500_2.10000V_0.00000T_Sep17-2014__21-16-02_001_091714.bin", "mod time(min)"=58230796.03333333, "file format"=enum."binary", "power(V)"=2.1, "Magn Field(T) "=0.0}, {"temperature"=14.976, "temperature str"="14.97600", "file path"=path "D:/Data/Ultrasound/LSCO/LSCO22__130814c/5_Cooling_2nd_try/September_2014/091714/14.97600K_500_2500_2.10000V_0.00000T_Sep17-2014__21-17-21_001_091714.bin", "last mod"=timestamp(3493847841 s since 1904-01-01), "file name str"="D:\\Data\\Ultrasound\\LSCO\\LSCO22__130814c\\5_Cooling_2nd_try\\September_2014\\091714\\14.97600K_500_2500_2.10000V_0.00000T_Sep17-2014__21-17-21_001_091714.bin", "mod time(min)"=58230797.35, "file format"=enum."binary", "power(V)"=2.1, "Magn Field(T) "=0.0}, {"temperature"=14.967, "temperature str"="14.96700", "file path"=path "D:/Data/Ultrasound/LSCO/LSCO22__130814c/5_Cooling_2nd_try/September_2014/091714/14.96700K_500_2500_2.10000V_0.00000T_Sep17-2014__21-18-40_001_091714.bin", "last mod"=timestamp(3493847920 s since 1904-01-01), "file name str"="D:\\Data\\Ultrasound\\LSCO\\LSCO22__130814c\\5_Cooling_2nd_try\\September_2014\\091714\\14.96700K_500_2500_2.10000V_0.00000T_Sep17-2014__21-18-40_001_091714.bin", "mod time(min)"=58230798.666666664, "file format"=enum."binary", "power(V)"=2.1, "Magn Field(T) "=0.0}, {"temperature"=14.967, "temperature str"="14.96700", "file path"=path "D:/Data/Ultrasound/LSCO/LSCO22__130814c/5_Cooling_2nd_try/September_2014/091714/14.96700K_500_2500_2.10000V_0.00000T_Sep17-2014__21-20-00_001_091714.bin", "last mod"=timestamp(3493848000 s since 1904-01-01), "file name str"="D:\\Data\\Ultrasound\\LSCO\\LSCO22__130814c\\5_Cooling_2nd_try\\September_2014\\091714\\14.96700K_500_2500_2.10000V_0.00000T_Sep17-2014__21-20-00_001_091714.bin", "mod time(min)"=58230800.0, "file format"=enum."binary", "power(V)"=2.1, "Magn Field(T) "=0.0}, {"temperature"=14.959, "temperature str"="14.95900", "file path"=path "D:/Data/Ultrasound/LSCO/LSCO22__130814c/5_Cooling_2nd_try/September_2014/091714/14.95900K_500_2500_2.10000V_0.00000T_Sep17-2014__21-21-19_001_091714.bin", 
